vi "Entities for Target.vi"(8 "error in (no error)":errorcluster, 10 "Target Name":string, 11 "Project Name":string) -> (0 "error out":errorcluster, 2 "Names":string[](array[string]), 3 "Entities":path[](array[path]))   [LabVIEW 2020, in "Conditum-Tools.lvlib" / "Entity Editor.lvclass"]
uses:
  Entity Editor.lvclass
  Entity Editor.lvclass/Entity Editor.ctl
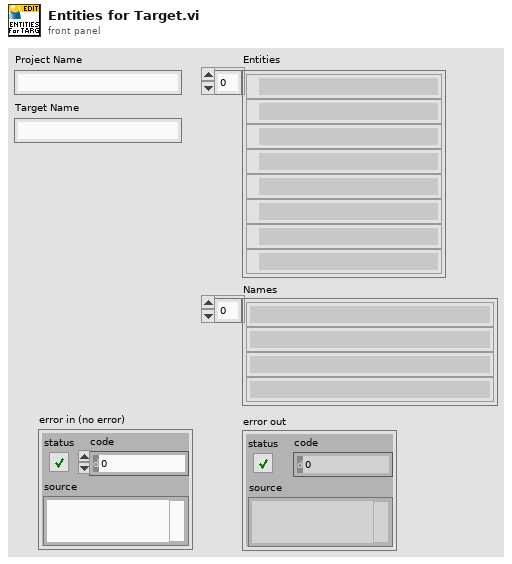
[diagram p1: front panel]
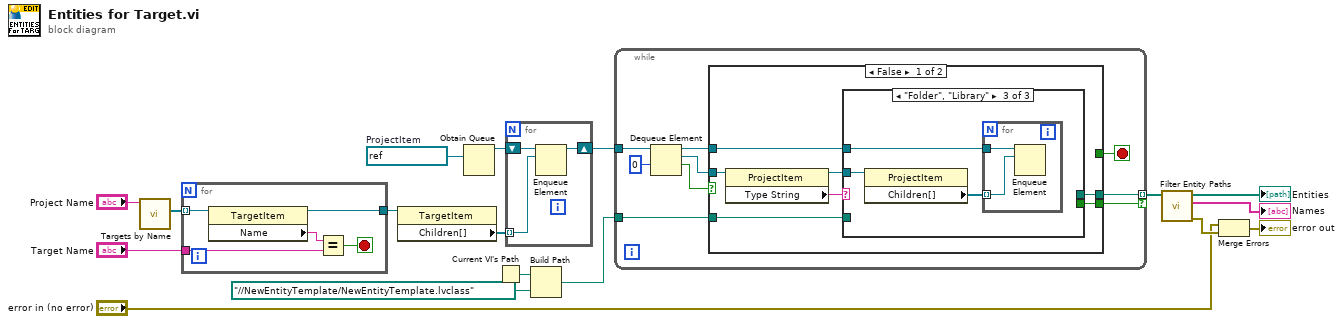
[diagram p0: block diagram]
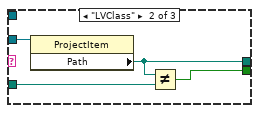
[diagram p3: hidden frame]
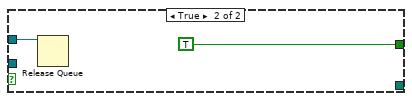
[diagram p4: hidden frame]
diagram:
  w13 = refnum<vi> refnum  # ProjectItem
  n1 = call "Targets by Name.vi"("Project Name"="Project Name") -> ("Targets"=w16:refnum<vi>[])  [unwired: 9 in, 1 out]
  n2 = for {
    tunnel: w16 -> [w22] mode=indexing
    tunnel: "Target Name" -> [w21]
    tunnel: [w19] -> w14
    stop <- w18 stop-if-true
    n3 = property class="TargetItem"(reference=w22) -> (reference out=w19:refnum<vi>, "Name"=w20:string)  [unwired: 1 in, 1 out]
    n4 = Equal?(x=w20, y=w21) -> (x = y?=w18:bool)
  }
  n5 = property class="TargetItem"(reference=w14) -> ("Children[]"=w12:refnum<vi>[])  [unwired: 1 in, 2 out]
  n6 = Obtain Queue(element data type=w13) -> (queue out=w11:refnum<queue>)  [unwired: 4 in, 2 out]
  n7 = Current VI's Path() -> (path=w8:path)
  n8 = for {
    tunnel: w12 -> [w24] mode=indexing
    shift-right: [w23] -> w10
    shift-left: w11 -> [w25]
    n9 = Enqueue Element(queue=w25, element=w24) -> (queue out=w23:refnum<queue>)  [unwired: 2 in, 2 out]
  }
  n10 = Build Path(base path=w8, name or relative path=path "../../NewEntityTemplate/NewEntityTemplate.lvclass" ("Relative Path from 1 to 2")) -> (appended path=w7:path)
  n11 = while {
    tunnel: w10 -> [w34]
    tunnel: w7 -> [w28]
    tunnel: [w27] -> w6 mode=indexing if=w26
    stop <- w29 stop-if-true
    n12 = Dequeue Element(queue=w34, timeout in ms (-1)=0) -> (queue out=w30:refnum<queue>, element=w31:refnum<vi>, timed out?=w32:bool)  [unwired: 1 in, 1 out]
    n13 = case shown="False" w32 {
      tunnel: w31 -> [w41 _]
      tunnel: w30 -> [w40 w52]
      tunnel: [_ TRUE] -> w29
      tunnel: w28 -> [w37 _]
      tunnel: [w36 _] -> w27
      tunnel: [w35 _] -> w26
      frame False {
        n14 = property class="ProjectItem"(reference=w41) -> (reference out=w38:refnum<vi>, "Type String"=w39:string)  [unwired: 1 in, 1 out]
        n15 = case shown="\"Folder\", \"Library\"" w39 {
          tunnel: w40 -> [_ _ w46]
          tunnel: w38 -> [_ w45 w48]
          tunnel: w37 -> [_ w44 _]
          tunnel: [_ w43 _] -> w36
          tunnel: [_ w42 _] -> w35
          frame Default {
          }
          frame "LVClass" {
            n16 = property class="ProjectItem"(reference=w45) -> ("Path"=w43:path)  [unwired: 1 in, 2 out]
            n17 = Not Equal?(x=w43, y=w44) -> (x != y?=w42:bool)
          }
          frame "Folder", "Library" {
            n18 = property class="ProjectItem"(reference=w48) -> ("Children[]"=w47:refnum<vi>[])  [unwired: 1 in, 2 out]
            n19 = for {
              tunnel: w47 -> [w49] mode=indexing
              tunnel: w46 -> [w50]
              n20 = Enqueue Element(queue=w50, element=w49) -> ()  [unwired: 2 in, 3 out]
            }
          }
        }
      }
      frame True {
        n21 = Release Queue(queue=w52) -> ()  [unwired: 2 in, 3 out]
      }
    }
  }
  n22 = call "Filter Entity Paths.vi"("Class Paths"=w6) -> ("error out"=w3:errorcluster, "Names"=→"Names":string[], "Entity Paths"=→"Entities":path[])  [unwired: 8 in]
  n23 = Merge Errors("error in (no error)", w3) -> (→"error out":errorcluster)
